vi "Read Base Description.vi"(11 "Mocha in":refnum<class "Milk.lvclass">) -> (2 "Description":string)   [LabVIEW 2013, in "Milk.lvclass"]
uses:
  Milk.lvclass
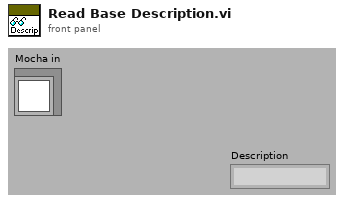
[diagram p1: front panel]
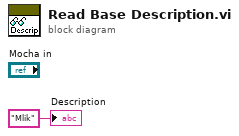
[diagram p0: block diagram]
diagram:
  "Description" <- "Mlik" ("string")
